vi "PLC-Reasembly.vi"(8 "error in":errorcluster, 11 "Reasembly data":T1) -> (0 "error out":errorcluster)   [LabVIEW 2016]
doc: "Go to PLC->SaveToDB action\n\nWabco 2017 All right reserved\nAuthor: maciej.szupienko@wabco-auto.com"
uses:
  PLC.CheckStatusReassembly.ctl
  PLC.Action.ctl
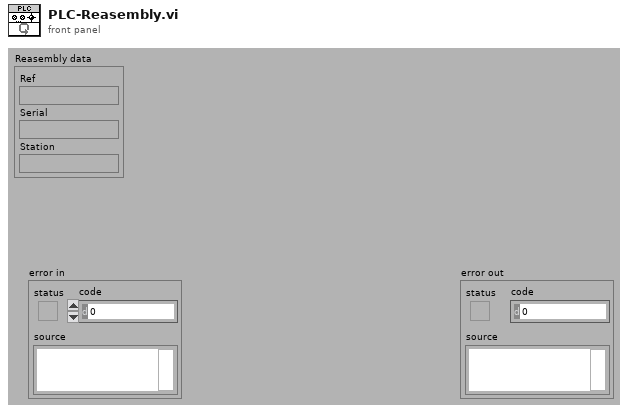
[diagram p1: front panel]
types:
  T1 = typedef "PLC.CheckStatusReassembly.ctl" = cluster{"Ref":string, "Serial":string, "Station":string}
  T2 = typedef "PLC.Action.ctl" = enum32{"idle", "constructor", "destructor", "-- PLC --", "Setup", "NewData", "ChangeOver", "CheckStatus", "Reasembly"}
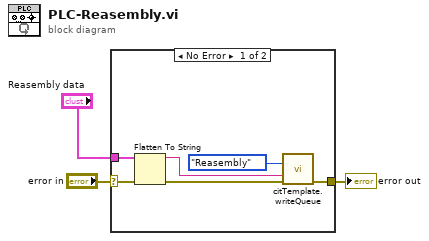
[diagram p0: block diagram]
diagram:
  n1 = case shown="No Error" "error in" {
    selector: "error in" -> [w9 w10]
    tunnel: [w8 w10] -> w2
    tunnel: "Reasembly data" -> [w5 _]
    frame No Error {
      n2 = Flatten To String(anything=w5, error in (no error)=w9) -> (data string=w4:string, error out=w6:errorcluster)  [unwired: 2 in, 1 out]
      n3 = call "citTemplate.writeQueue.vi"("event in (if not connected:all statemachine with data event)"=PLC.Action."Reasembly" ("Action"), "data in"=w4, "error in (no error)"=w6) -> ("error out"=w8:errorcluster)  [unwired: 12 in]
    }
    frame Error {
    }
  }
  "error out" <- w2
